vi "Read Version Info.vi"(7 "Unit ID (A)":string="A", 8 "error in":errorcluster, 11 "VISA Session In":refnum<visa-resource-name>="Alicat") -> (0 "error out":errorcluster, 1 "Software Sub-Rev":string, 2 "Software Rev":string, 3 "VISA Session Out":refnum<visa-resource-name>, 4 "Board Rev":string)   [LabVIEW 2023]
doc: "Reads the version info of the Alicat device. Returned values are the firmware/software version and sub-version, as well as the circuit board revision (if stored on the device). If the query is not supported, the returned values will be 1 for the software revision and 0 for the others."
uses:
  <vilib>/Instr/_visa.llb/VISA Flush IO Buffer Mask.ctl
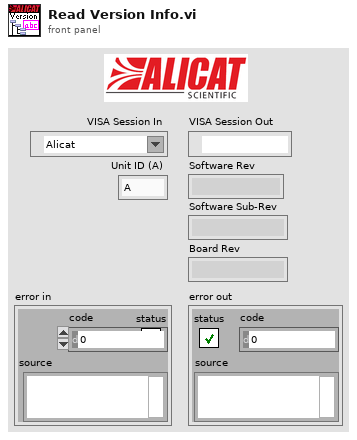
[diagram p1: front panel]
types:
  T1 = typedef "VISA Flush IO Buffer Mask.ctl" = u16
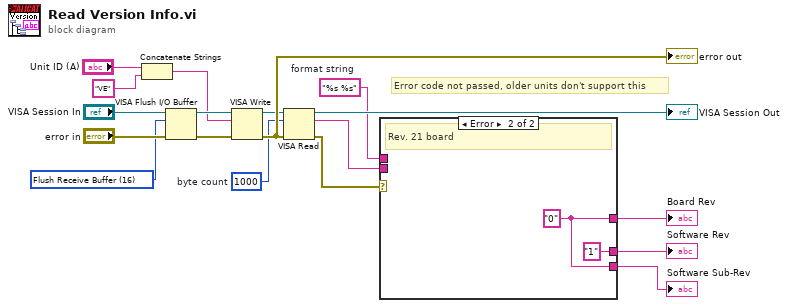
[diagram p0: block diagram]
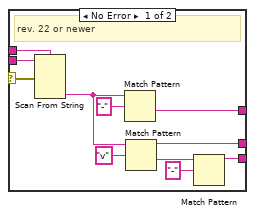
[diagram p2: hidden frame]
diagram:
  w14 = T1 16 items=["Flush Receive Buffer"=16, "Write Transmit Buffer to Device"=32, "Flush Receive Buffer (No I/O)"=64, "Flush Transmit Buffer"=128] ("Mask")
  w3 = "%s %s"  # format string
  w11 = u32 1000  # byte count
  # "Error code not passed, older units don't support this"
  n1 = Concatenate Strings("Unit ID (A)", "VE" ("string")) -> (w7:string)
  n2 = VISA Flush I/O Buffer(VISA resource name="VISA Session In", mask (16)=w14, error in (no error)="error in") -> (VISA resource name out=w16:refnum<visa-resource-name>, error out=w10:errorcluster)
  n3 = VISA Write(VISA resource name=w16, write buffer=w7, error in (no error)=w10) -> (VISA resource name out=w13:refnum<visa-resource-name>, error out=w18:errorcluster)  [unwired: 1 out]
  "error out" <- w18
  n4 = VISA Read(VISA resource name=w13, byte count=w11, error in (no error)=w18) -> (VISA resource name out=→"VISA Session Out":refnum<visa-resource-name>, read buffer=w2:string, error out=w1:errorcluster)  [unwired: 1 out]
  n5 = case shown="Error" w1 {
    selector: w1 -> [w20 _]
    tunnel: [w27 "1"] -> w6
    tunnel: [w25 w31] -> w5
    tunnel: [w23 w31] -> w4
    tunnel: w3 -> [w22 _]
    tunnel: w2 -> [w21 _]
    frame No Error {
      # "rev. 22 or newer"
      n6 = Scan From String(format string=w22, input string=w21, error in=w20) -> (output 2=w19:string)  [unwired: 4 in, 3 out]
      n7 = Match Pattern(string=w19, regular expression="-") -> (after substring=w25:string)  [unwired: 1 in, 3 out]
      n8 = Match Pattern(string=w19, regular expression="v") -> (before substring=w27:string, after substring=w24:string)  [unwired: 1 in, 2 out]
      n9 = Match Pattern(string=w24, regular expression="-") -> (before substring=w23:string)  [unwired: 1 in, 3 out]
    }
    frame Error {
      w31 = "0"
      # "Rev. 21 board"
    }
  }
  "Software Rev" <- w6
  "Software Sub-Rev" <- w4
  "Board Rev" <- w5
